vi "PickUpTote.vi"(8 "error in (no error)":errorcluster, 11 "JoystickDevRef":T1) -> ()   [LabVIEW 2014]
uses:
  <vilib>/Rock Robotics/WPI/Joystick/WPI_JoystickDevRef.ctl
  <vilib>/Rock Robotics/WPI/Joystick/WPI_JoystickDeviceEnum.ctl
  PickUpTote.ctl
  Gantry/GantryGlobals.vi
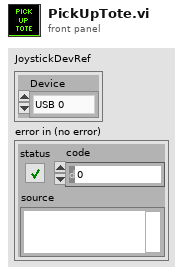
[diagram p1: front panel]
types:
  T1 = typedef "WPI_JoystickDevRef.ctl" = cluster{"Device":T2}
  T2 = typedef "WPI_JoystickDeviceEnum.ctl" = enum16{"USB 0", "USB 1", "USB 2", "USB 3", "USB 4", "USB 5"}
  T3 = typedef "PickUpTote.ctl" = enum16{"WaitForButtonPress", "ResetGanrty", "LowerLift", "CloseArms", "RaiseLiftOver1Tote", "RunRollers", "LowerLiftTo1Tote", "OpenArms"}
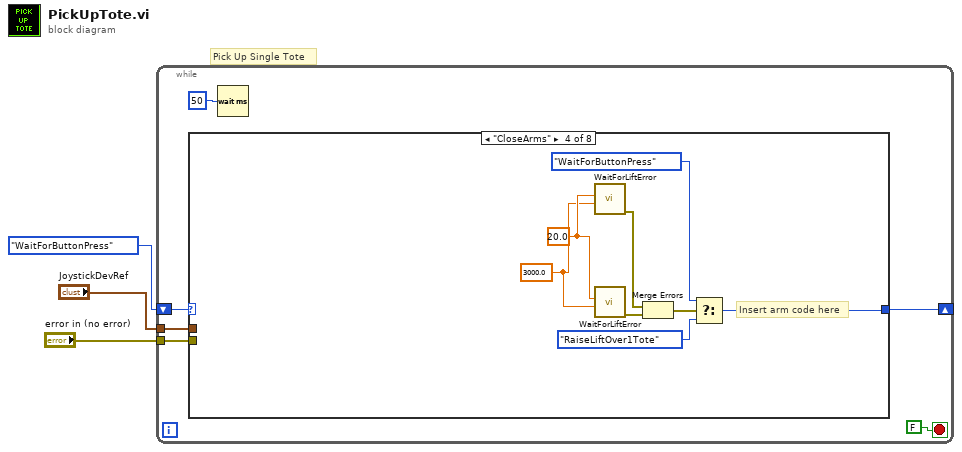
[diagram p0: block diagram]
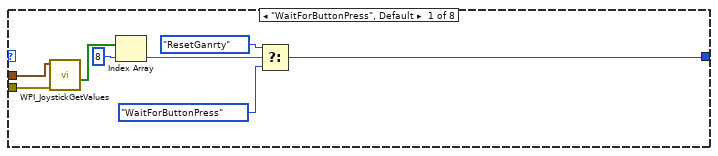
[diagram p2: hidden frame]
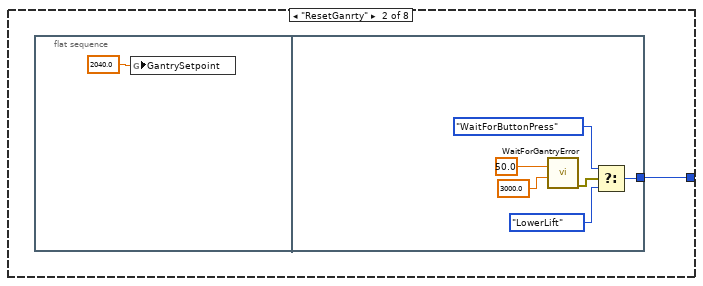
[diagram p3: hidden frame]
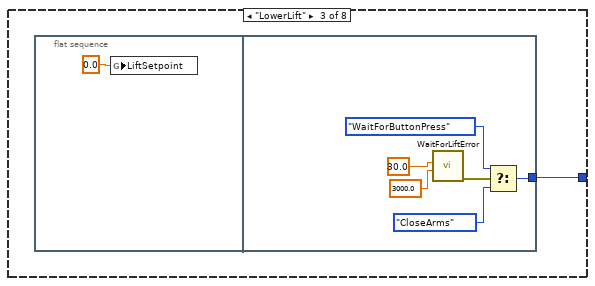
[diagram p4: hidden frame]
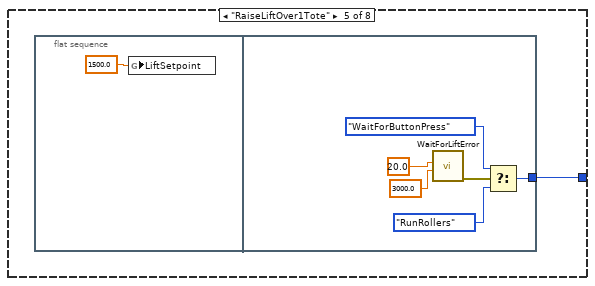
[diagram p5: hidden frame]
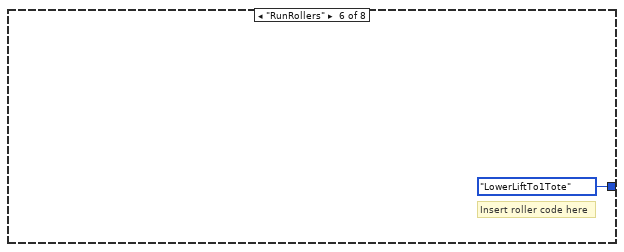
[diagram p6: hidden frame]
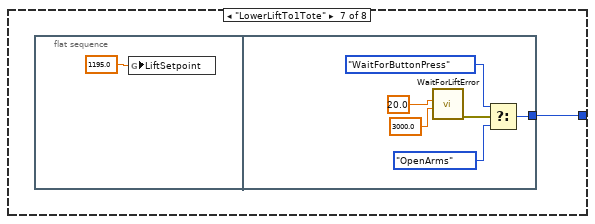
[diagram p7: hidden frame]
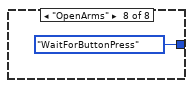
[diagram p8: hidden frame]
diagram:
  # "Pick Up Single Tote"
  n1 = while {
    shift-right: [w6] -> _
    shift-left: PickUpTote."WaitForButtonPress" ("Pick Up Tote") -> [w7]
    tunnel: "JoystickDevRef" -> [w5]
    tunnel: "error in (no error)" -> [w4]
    stop <- FALSE stop-if-true
    n2 = case shown="\"CloseArms\"" w7 {
      tunnel: [w14 w18 w26 w35 w42 PickUpTote."LowerLiftTo1Tote" ("Pick Up Tote") w51 PickUpTote."WaitForButtonPress" ("Pick Up Tote")] -> w6
      tunnel: w5 -> [w11 _ _ _ _ _ _ _]
      tunnel: w4 -> [w10 _ _ _ _ _ _ _]
      frame "WaitForButtonPress", Default {
        n3 = call <vilib>:"WPI_JoystickGetValues.vi"("error in (no error)"=w10, "JoystickDevRef"=w11) -> ("Buttons"=w12:bool[])  [unwired: 5 in, 4 out]
        n4 = Index Array(array=w12, index=8) -> (element=w13:bool)
        n5 = Select(t=PickUpTote."ResetGanrty" ("Pick Up Tote"), s=w13, f=PickUpTote."WaitForButtonPress" ("Pick Up Tote")) -> (s? t:f=w14:T3)
      }
      frame "ResetGanrty" {
        n6 = flat-sequence {
          tunnel: [w23] -> w18
          frame #0 {
            n7 = global write "GantryGlobals.vi" "GantrySetpoint"(2040.0 ("GantryError")) -> ()
          }
          frame #1 {
            n8 = call "WaitForGantryError.vi"("Timeout (ms)"=3000.0, "AllowedError"=50.0 ("Error")) -> ("error out"=w22:errorcluster)  [unwired: 9 in]
            n9 = Select(t=PickUpTote."WaitForButtonPress" ("Pick Up Tote"), s=w22, f=PickUpTote."LowerLift" ("Pick Up Tote")) -> (s? t:f=w23:T3)
          }
        }
      }
      frame "LowerLift" {
        n10 = flat-sequence {
          tunnel: [w28] -> w26
          frame #0 {
            n11 = global write "GantryGlobals.vi" "LiftSetpoint"(0.0 ("LiftSetpoint")) -> ()
          }
          frame #1 {
            n12 = call "WaitForLiftError.vi"("Timeout (ms)"=3000.0, "AllowedError"=30.0 ("Error")) -> ("error out"=w30:errorcluster)  [unwired: 9 in]
            n13 = Select(t=PickUpTote."WaitForButtonPress" ("Pick Up Tote"), s=w30, f=PickUpTote."CloseArms" ("Pick Up Tote")) -> (s? t:f=w28:T3)
          }
        }
      }
      frame "CloseArms" {
        w34 = 3000.0 ("Timeout (ms)")
        w41 = 20.0
        # "Insert arm code here"
        n14 = call "WaitForLiftError.vi"("Timeout (ms)"=w34, "AllowedError"=w41) -> ("error out"=w40:errorcluster)  [unwired: 9 in]
        n15 = call "WaitForLiftError.vi"("Timeout (ms)"=w34, "AllowedError"=w41) -> ("error out"=w39:errorcluster)  [unwired: 9 in]
        n16 = Merge Errors(w40, w39) -> (w38:errorcluster)
        n17 = Select(t=PickUpTote."WaitForButtonPress" ("Pick Up Tote"), s=w38, f=PickUpTote."RaiseLiftOver1Tote" ("Pick Up Tote")) -> (s? t:f=w35:T3)
      }
      frame "RaiseLiftOver1Tote" {
        n18 = flat-sequence {
          tunnel: [w47] -> w42
          frame #0 {
            n19 = global write "GantryGlobals.vi" "LiftSetpoint"(1500.0 ("LiftSetpoint")) -> ()
          }
          frame #1 {
            n20 = call "WaitForLiftError.vi"("Timeout (ms)"=3000.0, "AllowedError"=20.0 ("Error")) -> ("error out"=w44:errorcluster)  [unwired: 9 in]
            n21 = Select(t=PickUpTote."WaitForButtonPress" ("Pick Up Tote"), s=w44, f=PickUpTote."RunRollers" ("Pick Up Tote")) -> (s? t:f=w47:T3)
          }
        }
      }
      frame "RunRollers" {
        # "Insert roller code here"
      }
      frame "LowerLiftTo1Tote" {
        n22 = flat-sequence {
          tunnel: [w54] -> w51
          frame #0 {
            n23 = global write "GantryGlobals.vi" "LiftSetpoint"(1195.0 ("GantrySetpoint")) -> ()
          }
          frame #1 {
            n24 = call "WaitForLiftError.vi"("Timeout (ms)"=3000.0, "AllowedError"=20.0 ("Error")) -> ("error out"=w53:errorcluster)  [unwired: 9 in]
            n25 = Select(t=PickUpTote."WaitForButtonPress" ("Pick Up Tote"), s=w53, f=PickUpTote."OpenArms" ("Pick Up Tote")) -> (s? t:f=w54:T3)
          }
        }
      }
      frame "OpenArms" {
      }
    }
    n26 = Wait (ms)(milliseconds to wait=u32 50) -> ()  [unwired: 1 out]
  }
